vi "ClosePython.vi"(8 "error in (no error)":errorcluster caption="entrée d'erreur (pas d'erreur)", 11 "Scikit-learn en entrée":refnum<class "Scikit-learn.lvclass">) -> (0 "error out":errorcluster caption="sortie d'erreur", 3 "Scikit-learn en sortie":refnum<class "Scikit-learn.lvclass">)   [LabVIEW 2020, in "Scikit-learn.lvclass"]
doc: "Close properly reference to release memory"
uses:
  Scikit-learn.lvclass
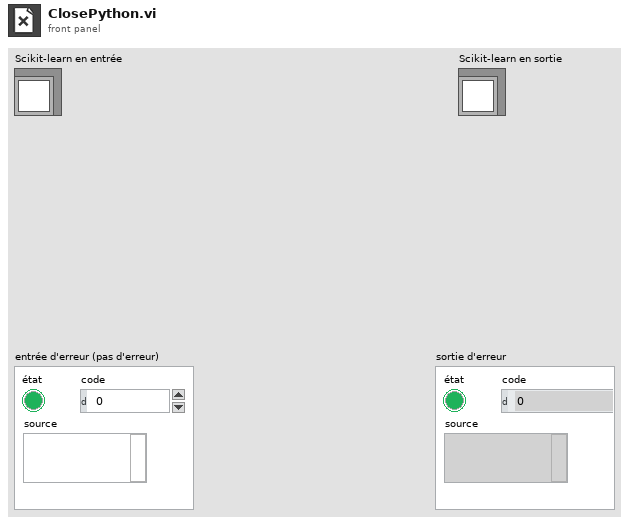
[diagram p1: front panel]
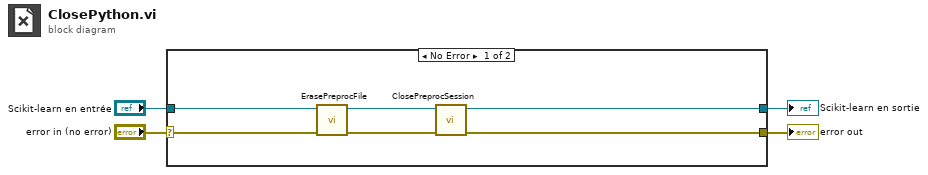
[diagram p0: block diagram]
diagram:
  n1 = case shown="No Error" "error in (no error)" {
    selector: "error in (no error)" -> [w9 w12]
    tunnel: [w5 w12] -> w3
    tunnel: [w6 w11] -> w1
    tunnel: "Scikit-learn en entrée" -> [w10 w11]
    frame No Error {
      n2 = call-dynamic "ErasePreprocFile.vi"("error in (no error)"=w9, "Python in"=w10) -> ("error out"=w7:errorcluster, "Python out"=w8:refnum<class "Scikit-learn.lvclass">)  [unwired: 8 in]
      n3 = call-dynamic "ClosePreprocSession.vi"("error in (no error)"=w7, "Python in"=w8) -> ("error out"=w5:errorcluster, "Python out"=w6:refnum<class "Scikit-learn.lvclass">)  [unwired: 8 in]
    }
    frame Error {
    }
  }
  "error out" <- w3
  "Scikit-learn en sortie" <- w1
